vi "Process Data1D.vi"(8 "error in (no error)":errorcluster, 10 "Data1D in":refnum<class "Data1D.lvclass">, 11 "AbstractProcessor1D in":refnum<class "AbstractProcessor1D.lvclass">) -> (0 "error out":errorcluster, 2 "Data1D out":refnum<class "Data1D.lvclass">, 3 "AbstractProcessor1D out":refnum<class "AbstractProcessor1D.lvclass">)   [LabVIEW 2014, in "AbstractProcessor1D.lvclass"]
uses:
  AbstractProcessor1D.lvclass
  Model/Data/Data1D/Data1D.lvclass
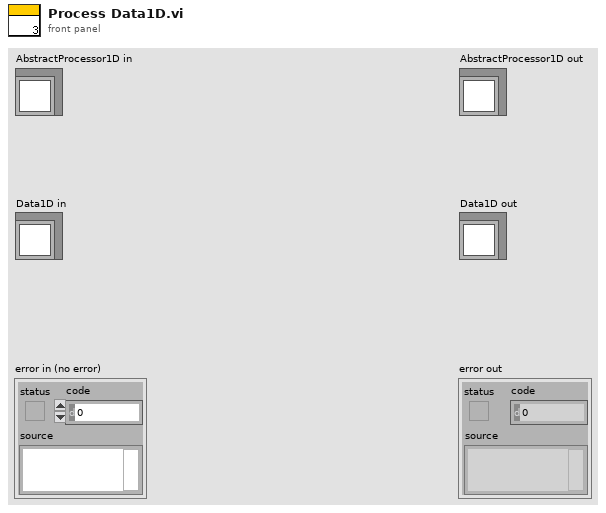
[diagram p1: front panel]
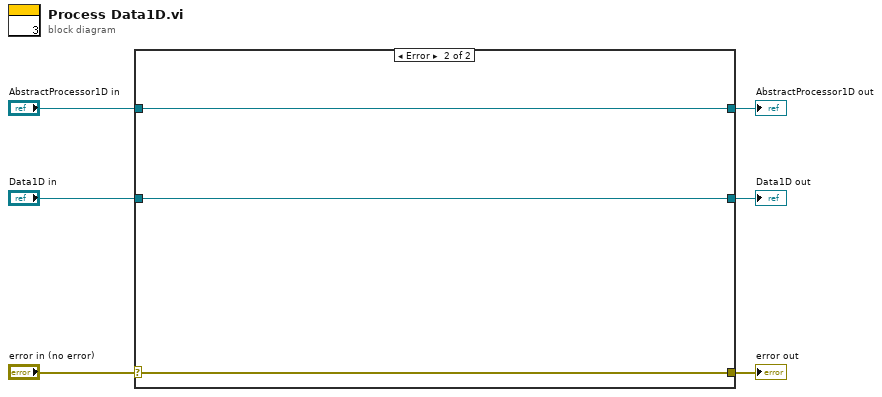
[diagram p0: block diagram]
diagram:
  n1 = case shown="Error" "error in (no error)" {
    selector: "error in (no error)" -> [w8 w12]
    tunnel: [w8 w12] -> w5
    tunnel: [w9 w11] -> w3
    tunnel: "AbstractProcessor1D in" -> [w9 w11]
    tunnel: [w7 w10] -> w2
    tunnel: "Data1D in" -> [w7 w10]
    frame No Error {
      # "Wire the error cluster across even in the \"No Error\"\ncase so that warnings get propagated."
    }
    frame Error {
    }
  }
  "error out" <- w5
  "AbstractProcessor1D out" <- w3
  "Data1D out" <- w2
